vi "test_libssh2_channel_window_read_ex.vi"() -> ()   [LabVIEW 2013, in "libssh2_integration_tests.lvlib"]
uses:
  libssh2_integration_tests.lvlib
  <vilib>/addons/_JKI Toolkits/Caraya/classes/Test/Test.lvclass
  libssh2/libssh2.lvlib
  <vilib>/addons/_JKI Toolkits/Caraya/classes/Assert/Assert.lvclass
panel:
  out "error out":errorcluster
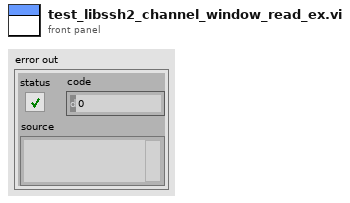
[diagram p1: front panel]
types:
  T1 = typedef "libssh2.lvlib/Session Refnum.ctl" = refnum<k1>
  T2 = typedef "libssh2.lvlib/Channel Refnum.ctl" = refnum<k1>
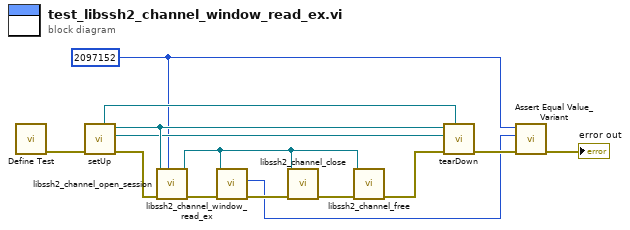
[diagram p0: block diagram]
diagram:
  w2 = u32 2097152 ("window_size (2 MiB)")
  n1 = call <vilib>:"Define Test.vi"() -> ("error out"=w13:errorcluster)  [unwired: 10 in, 1 out]
  n2 = call "setUp.vi"("error in (no error)"=w13) -> ("error out"=w6:errorcluster, "connection ID"=w9:refnum<k5>, "session"=w10:T1, "fixture"=w11:refnum<class "Server Fixture.lvclass">)  [unwired: 7 in]
  n3 = call "libssh2_channel_open_session.vi"("window_size (2 MiB)"=w2, "error in (no error)"=w6, "session"=w10) -> ("error out"=w3:errorcluster, "channel"=w7:T2)  [unwired: 7 in]
  n4 = call "libssh2_channel_window_read_ex.vi"("error in (no error)"=w3, "channel"=w7) -> ("error out"=w4:errorcluster, "initial window size"=w1:u32)  [unwired: 6 in, 2 out]
  n5 = call "libssh2_channel_close.vi"("error in (no error)"=w4, "channel"=w7) -> ("error out"=w8:errorcluster)  [unwired: 9 in]
  n6 = call "libssh2_channel_free.vi"("error in (no error)"=w8, "channel"=w7) -> ("error out"=w5:errorcluster)  [unwired: 9 in]
  n7 = call "tearDown.vi"("fixture"=w11, "error in (no error)"=w5, "connection ID"=w9, "session"=w10) -> ("error out"=w12:errorcluster)  [unwired: 7 in]
  n8 = call <vilib>:"Assert Equal Value_Variant.vi"("error in (no error)"=w12, "Y"=w1, "X"=w2) -> ("error out"=→"error out":errorcluster)  [unwired: 7 in, 1 out]
